vi "PH_Beckhoff-16BB_Testtool.panel.vi"(0 "object ref":refnum<vi>, 5 "error in (no error)":errorcluster) -> (19 "error out":errorcluster)   [LabVIEW 2014, in "PH_Beckhoff-16BB_Testtool.lvlib"]
doc: "By this VI a ross relais can be monitored and switched. \n\nThe indicators \"CLOSED\", \"OPEN\" and \"SWITCH STATE\" show the value of the Beckhoff-Tag: blue indicates bad tag status reference problems, darkgreen false and lightgreen on. If everything is working fine, \"CLOSED\" and \"SWITCH STATE\" should show the same value, while \"OPEN\" has the opposite value. \n\nThe oval button switches the ross relais. It should be in the same state as the \"SWITCH STATE\" indicator. \n\n\"EXIT\" closes the front panel (GUI), while \"Delete Instance\" disconnects and removes the instance from the PCS.\n\nThis VI has no machine safety relevant logig: there is neither a check of internal conclict nor with other objects, for example conflict with other ross relais. Therefore it must be handled with care and should be operated by well educated operators only. It is forseen exclusively for direct operating and testing of the system. \n\nLicense Agreement for this software:\n\nCopyright (C)\nGesellschaft für Schwerionenforschung, GSI\nPlanckstr. 1\n64291 Darmstadt\nGermany\n\nContact: D.Beck@gsi.de \n\nThis program is free software; you can redistribute it and/or modify it under the terms of the GNU General Public License as published by the Free Software Foundation; either version 2 of the license, or (at your option) any later version.\n\nThis program is distributed in the hope that it will be useful, but WITHOUT ANYW ARRANTY; without even the implied warranty of MERCHANTABILITY or FITNESS FOR A PARTICULAR PURPOSE. See the GNU General License for more details (http://www.gnu.org).\n\nGesellschaft für Schwerionenforschung, GSI\nPlanckstr. 1, 64291 Darmstadt, Germany\nFor all questions and ideas contact: M.Richter@gsi.de, H.Brand@gsi.de or D.Beck@gsi.de.\nLast update: 18-DEC-2002"
uses:
  PH_Beckhoff-16BB_Testtool.lvlib
  CS_Core/CSSystem/CoreLib/CoreLib.short 2 byte array.vi
  CS_Core/CSSystem/CoreLib/CoreLib.string 2 byte array.vi
  PH_Basics/PH_Common/PH_Common.lvlib
  CS_Core/BaseProcess/BaseProcess.lvlib
  CS_Core/CSSystem/CoreLib/CoreLib.lvlib
  PH_Basics/PH_Class/PH_Class.lvlib
panel:
  out "Instance":string
  out "_DC_int_ok":u32(colorbox) caption="POWER Int"
  in  "Move in 16":bool caption="Dir"
  in  "Move 16":bool caption="Move"
  out "_BB_16_remote_controlled":u32(colorbox) caption="REMOTE"
  out "_BB_16_out":u32(colorbox) caption="OUT"
  out "_BB_16_in":u32(colorbox) caption="IN"
  out "_BB_16_move":u32(colorbox) caption="MOVE"
  out "_BB_16_move_in":u32(colorbox) caption="MOVE IN"
  in  "Move in 15":bool caption="Dir"
  in  "Move 15":bool caption="Move"
  out "_BB_15_remote_controlled":u32(colorbox) caption="REMOTE"
  out "_BB_15_out":u32(colorbox) caption="OUT"
  out "_BB_15_in":u32(colorbox) caption="IN"
  out "_BB_15_move":u32(colorbox) caption="MOVE"
  out "_BB_15_move_in":u32(colorbox) caption="MOVE IN"
  in  "Move in 14":bool caption="Dir"
  in  "Move 14":bool caption="Move"
  out "_BB_14_remote_controlled":u32(colorbox) caption="REMOTE"
  out "_BB_14_out":u32(colorbox) caption="OUT"
  out "_BB_14_in":u32(colorbox) caption="IN"
  out "_BB_14_move":u32(colorbox) caption="MOVE"
  out "_BB_14_move_in":u32(colorbox) caption="MOVE IN"
  in  "Move in 13":bool caption="Dir"
  in  "Move 13":bool caption="Move"
  out "_BB_13_remote_controlled":u32(colorbox) caption="REMOTE"
  out "_BB_13_out":u32(colorbox) caption="OUT"
  out "_BB_13_in":u32(colorbox) caption="IN"
  out "_BB_13_move":u32(colorbox) caption="MOVE"
  out "_BB_13_move_in":u32(colorbox) caption="MOVE IN"
  in  "Move in 12":bool caption="Dir"
  in  "Move 12":bool caption="Move"
  out "_BB_12_remote_controlled":u32(colorbox) caption="REMOTE"
  out "_BB_12_out":u32(colorbox) caption="OUT"
  out "_BB_12_in":u32(colorbox) caption="IN"
  out "_BB_12_move":u32(colorbox) caption="MOVE"
  out "_BB_12_move_in":u32(colorbox) caption="MOVE IN"
  in  "Move in 11":bool caption="Dir"
  in  "Move 11":bool caption="Move"
  out "_BB_11_remote_controlled":u32(colorbox) caption="REMOTE"
  out "_BB_11_out":u32(colorbox) caption="OUT"
  out "_BB_11_in":u32(colorbox) caption="IN"
  out "_BB_11_move":u32(colorbox) caption="MOVE"
  out "_BB_11_move_in":u32(colorbox) caption="MOVE IN"
  in  "Move in 10":bool caption="Dir"
  in  "Move 10":bool caption="Move"
  out "_BB_10_remote_controlled":u32(colorbox) caption="REMOTE"
  out "_BB_10_out":u32(colorbox) caption="OUT"
  out "_BB_10_in":u32(colorbox) caption="IN"
  out "_BB_10_move":u32(colorbox) caption="MOVE"
  out "_BB_10_move_in":u32(colorbox) caption="MOVE IN"
  in  "Move in 9":bool caption="Dir"
  in  "Move 9":bool caption="Move"
  out "_BB_9_remote_controlled":u32(colorbox) caption="REMOTE"
  out "_BB_9_out":u32(colorbox) caption="OUT"
  out "_BB_9_in":u32(colorbox) caption="IN"
  out "_BB_9_move":u32(colorbox) caption="MOVE"
  out "_BB_9_move_in":u32(colorbox) caption="MOVE IN"
  in  "Move in 8":bool caption="Dir"
  in  "Move 8":bool caption="Move"
  out "_BB_8_remote_controlled":u32(colorbox) caption="REMOTE"
  out "_BB_8_out":u32(colorbox) caption="OUT"
  out "_BB_8_in":u32(colorbox) caption="IN"
  out "_BB_8_move":u32(colorbox) caption="MOVE"
  out "_BB_8_move_in":u32(colorbox) caption="MOVE IN"
  in  "Move in 7":bool caption="Dir"
  in  "Move 7":bool caption="Move"
  out "_BB_7_remote_controlled":u32(colorbox) caption="REMOTE"
  out "_BB_7_out":u32(colorbox) caption="OUT"
  out "_BB_7_in":u32(colorbox) caption="IN"
  out "_BB_7_move":u32(colorbox) caption="MOVE"
  out "_BB_7_move_in":u32(colorbox) caption="MOVE IN"
  in  "Move in 6":bool caption="Dir"
  in  "Move 6":bool caption="Move"
  out "_BB_6_remote_controlled":u32(colorbox) caption="REMOTE"
  out "_BB_6_out":u32(colorbox) caption="OUT"
  out "_BB_6_in":u32(colorbox) caption="IN"
  out "_BB_6_move":u32(colorbox) caption="MOVE"
  out "_BB_6_move_in":u32(colorbox) caption="MOVE IN"
  in  "Move in 5":bool caption="Dir"
  in  "Move 5":bool caption="Move"
  out "_BB_5_remote_controlled":u32(colorbox) caption="REMOTE"
  out "_BB_5_out":u32(colorbox) caption="OUT"
  out "_BB_5_in":u32(colorbox) caption="IN"
  out "_BB_5_move":u32(colorbox) caption="MOVE"
  out "_BB_5_move_in":u32(colorbox) caption="MOVE IN"
  in  "Move in 4":bool caption="Dir"
  in  "Move 4":bool caption="Move"
  out "_BB_4_remote_controlled":u32(colorbox) caption="REMOTE"
  out "_BB_4_out":u32(colorbox) caption="OUT"
  out "_BB_4_in":u32(colorbox) caption="IN"
  out "_BB_4_move":u32(colorbox) caption="MOVE"
  out "_BB_4_move_in":u32(colorbox) caption="MOVE IN"
  in  "Move in 3":bool caption="Dir"
  in  "Move 3":bool caption="Move"
  out "_BB_3_remote_controlled":u32(colorbox) caption="REMOTE"
  out "_BB_3_out":u32(colorbox) caption="OUT"
  out "_BB_3_in":u32(colorbox) caption="IN"
  out "_BB_3_move":u32(colorbox) caption="MOVE"
  out "_BB_3_move_in":u32(colorbox) caption="MOVE IN"
  in  "Move in 2":bool caption="Dir"
  in  "Move 2":bool caption="Move"
  out "_BB_2_remote_controlled":u32(colorbox) caption="REMOTE"
  out "_BB_2_out":u32(colorbox) caption="OUT"
  out "_BB_2_in":u32(colorbox) caption="IN"
  out "_BB_2_move":u32(colorbox) caption="MOVE"
  out "_BB_2_move_in":u32(colorbox) caption="MOVE IN"
  out "_DC_ext_ok":u32(colorbox) caption="POWER Ext"
  in  "Move in 1":bool caption="Dir"
  in  "Move 1":bool caption="Move"
  out "_BB_1_remote_controlled":u32(colorbox) caption="REMOTE"
  out "_BB_1_out":u32(colorbox) caption="OUT"
  out "_BB_1_in":u32(colorbox) caption="IN"
  out "_BB_1_move":u32(colorbox) caption="MOVE"
  out "_BB_1_move_in":u32(colorbox) caption="MOVE IN"
  in  "Delete":bool
  # "PCS"
  # "3.40"
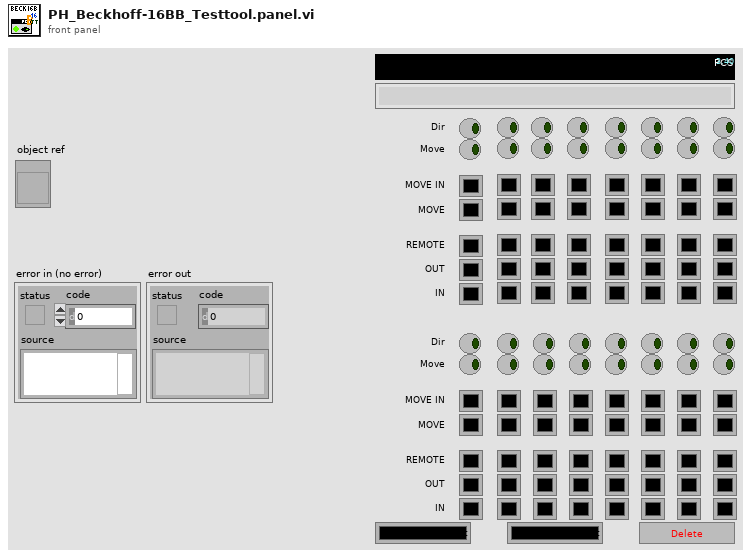
[diagram p1: front panel]
types:
  T1 = typedef "PH_Beckhoff-16BB_Testtool.lvlib/PH_Beckhoff-16BB_Testtool.i attribute.ctl" = cluster{"GUI Refs":refnum<vi>[], "16BB Instance":string}
  T2 = typedef "CoreDefs.rawDataType.ctl" = i8[]
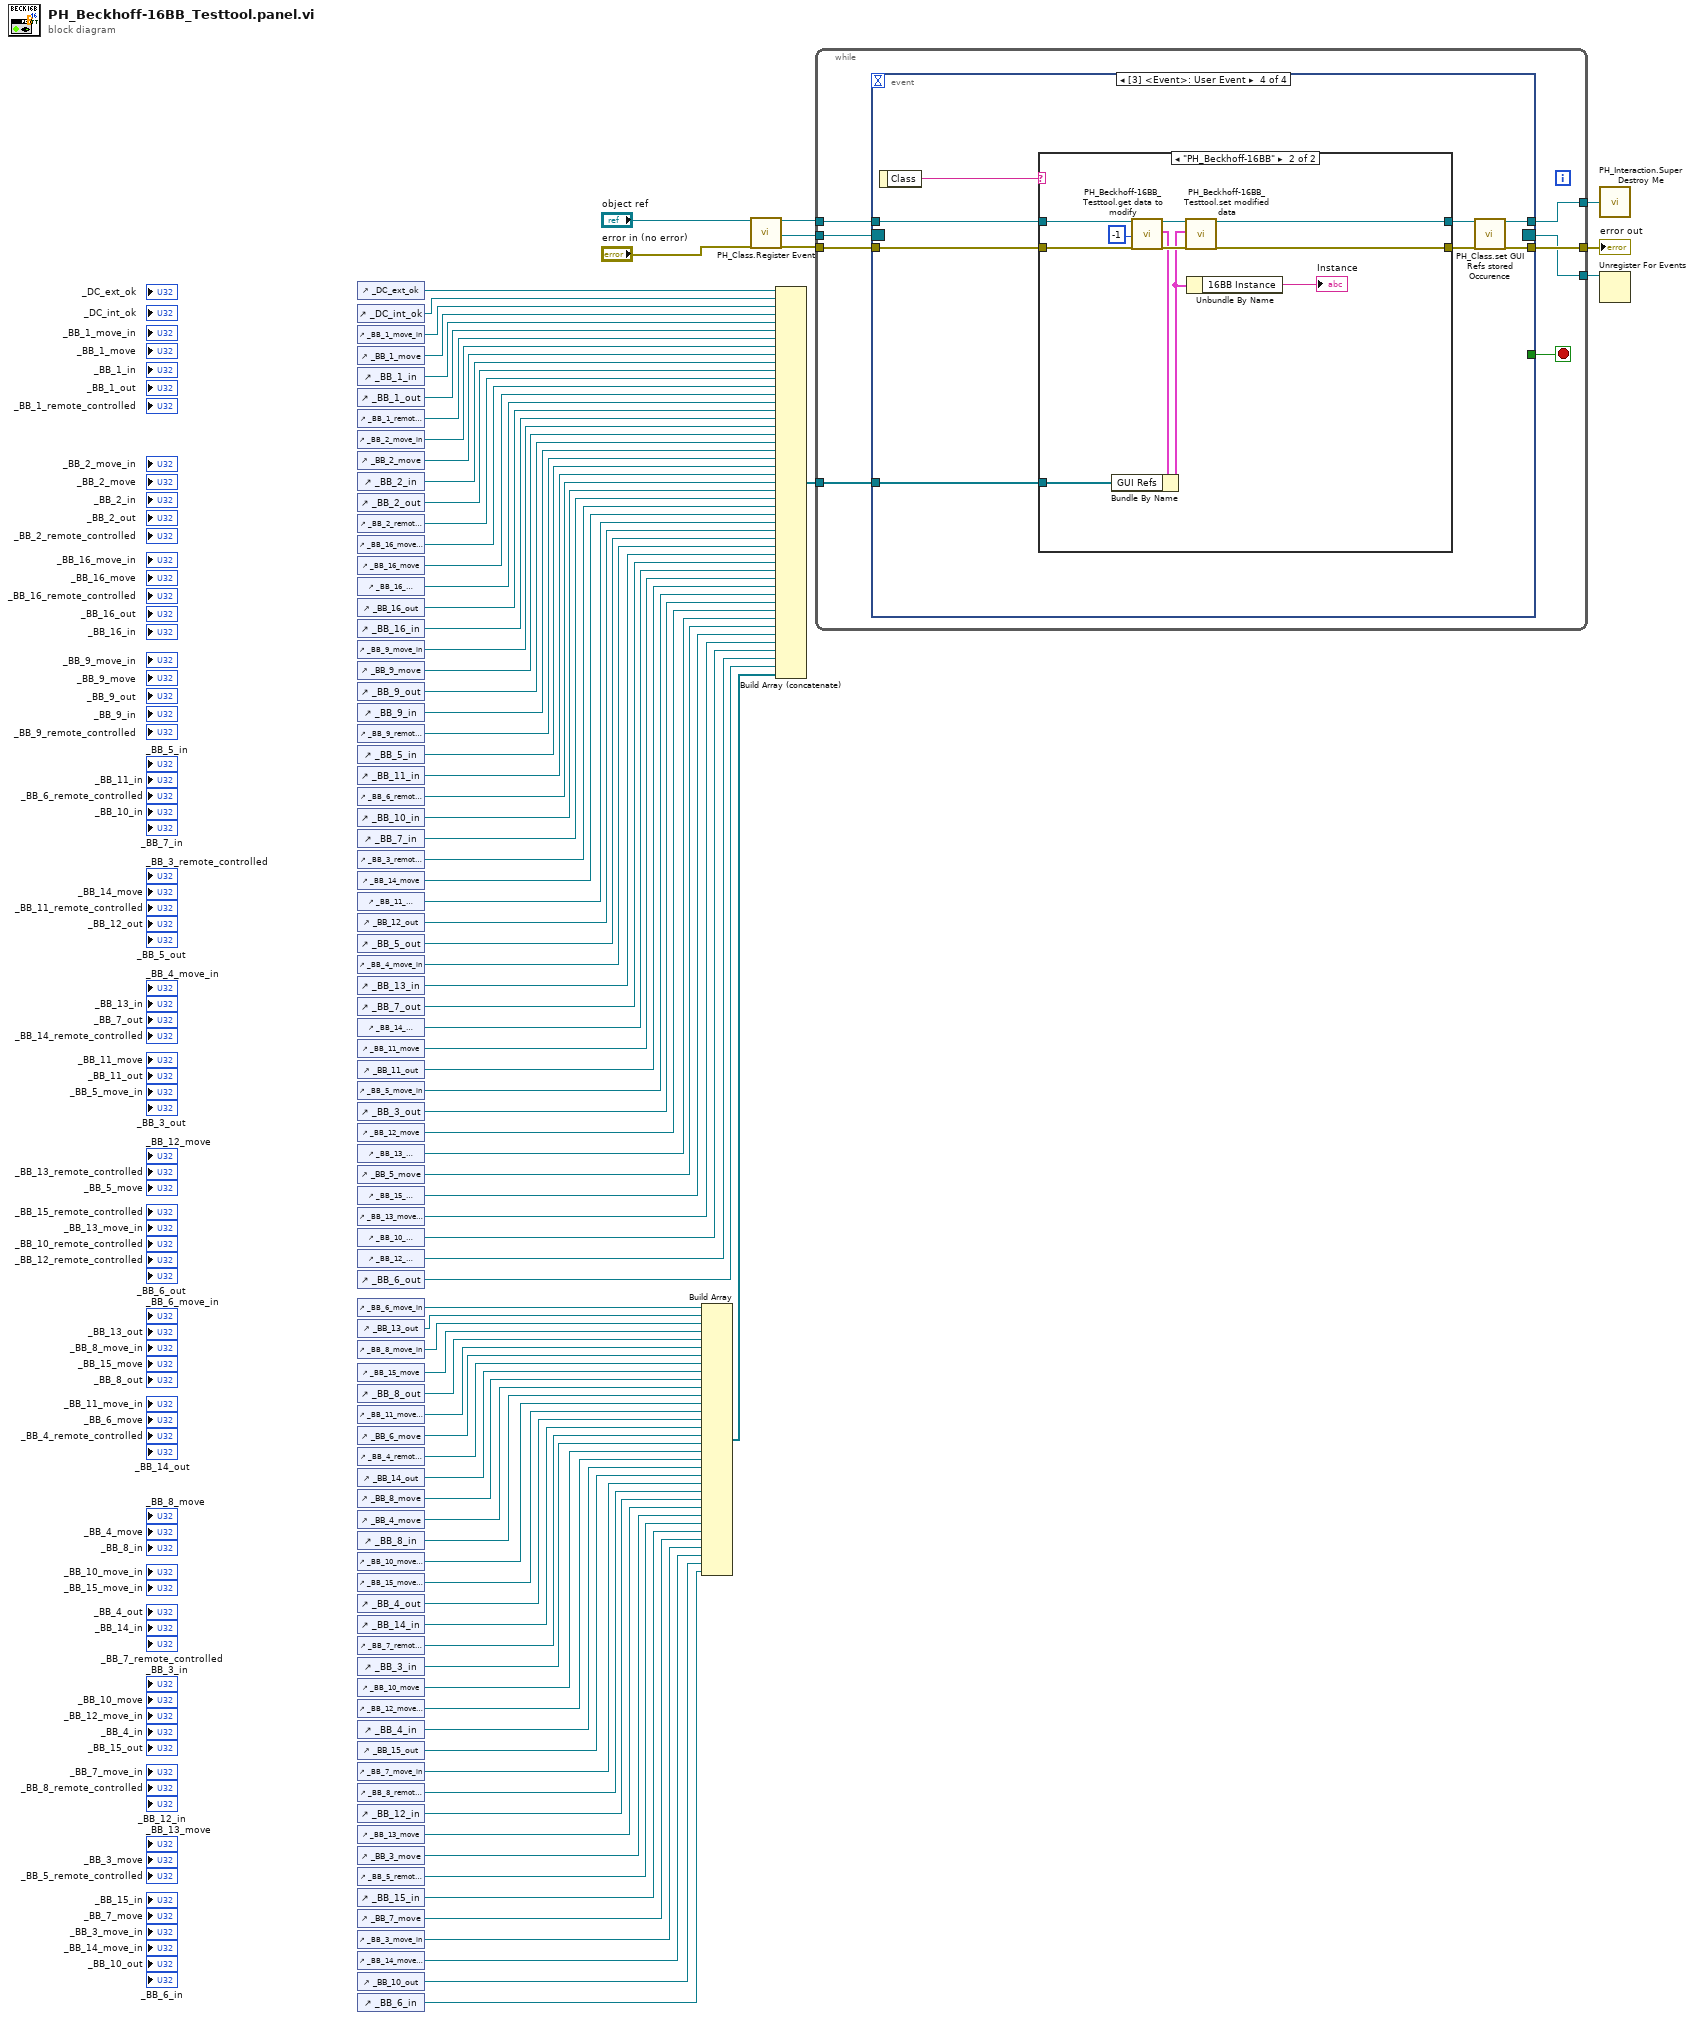
[diagram p0: block diagram]
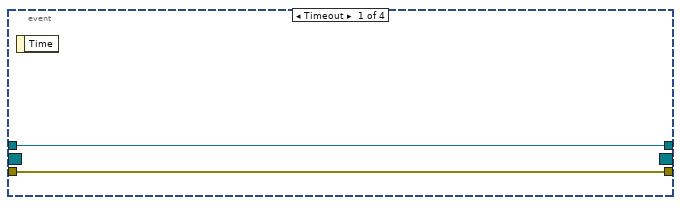
[diagram p2: hidden frame]
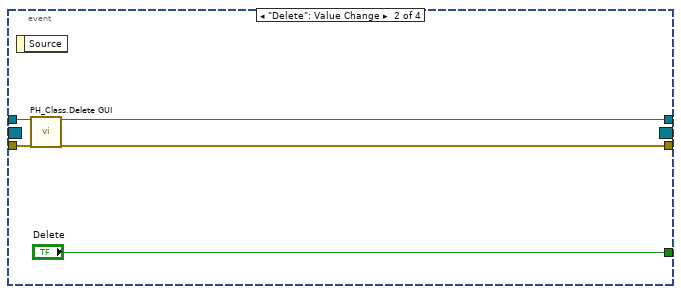
[diagram p3: hidden frame]
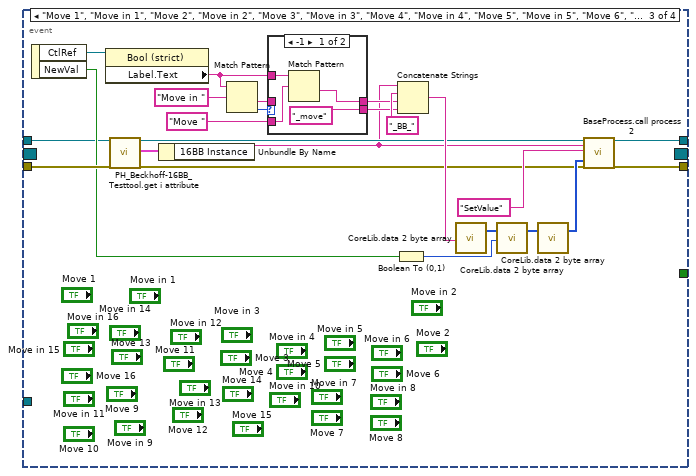
[diagram p4: hidden frame]
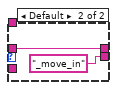
[diagram p5: hidden frame]
diagram:
  n1 = control-ref of="_DC_ext_ok"() -> (w84:refnum<vi>)
  n2 = control-ref of="_DC_int_ok"() -> (w85:refnum<vi>)
  n3 = control-ref of="_BB_1_move_in"() -> (w90:refnum<vi>)
  n4 = control-ref of="_BB_1_move"() -> (w89:refnum<vi>)
  n5 = control-ref of="_BB_1_in"() -> (w88:refnum<vi>)
  n6 = control-ref of="_BB_1_out"() -> (w87:refnum<vi>)
  n7 = control-ref of="_BB_1_remote_controlled"() -> (w86:refnum<vi>)
  n8 = control-ref of="_BB_2_move_in"() -> (w83:refnum<vi>)
  n9 = control-ref of="_BB_2_move"() -> (w82:refnum<vi>)
  n10 = control-ref of="_BB_2_in"() -> (w81:refnum<vi>)
  n11 = control-ref of="_BB_2_out"() -> (w80:refnum<vi>)
  n12 = control-ref of="_BB_2_remote_controlled"() -> (w79:refnum<vi>)
  n13 = control-ref of="_BB_16_move_in"() -> (w78:refnum<vi>)
  n14 = control-ref of="_BB_16_move"() -> (w77:refnum<vi>)
  n15 = control-ref of="_BB_16_remote_controlled"() -> (w76:refnum<vi>)
  n16 = control-ref of="_BB_16_out"() -> (w75:refnum<vi>)
  n17 = control-ref of="_BB_16_in"() -> (w74:refnum<vi>)
  n18 = control-ref of="_BB_9_move_in"() -> (w73:refnum<vi>)
  n19 = control-ref of="_BB_9_move"() -> (w72:refnum<vi>)
  n20 = control-ref of="_BB_9_out"() -> (w71:refnum<vi>)
  n21 = control-ref of="_BB_9_in"() -> (w70:refnum<vi>)
  n22 = control-ref of="_BB_9_remote_controlled"() -> (w69:refnum<vi>)
  n23 = control-ref of="_BB_5_in"() -> (w68:refnum<vi>)
  n24 = control-ref of="_BB_11_in"() -> (w67:refnum<vi>)
  n25 = control-ref of="_BB_6_remote_controlled"() -> (w66:refnum<vi>)
  n26 = control-ref of="_BB_10_in"() -> (w65:refnum<vi>)
  n27 = control-ref of="_BB_7_in"() -> (w64:refnum<vi>)
  n28 = control-ref of="_BB_3_remote_controlled"() -> (w63:refnum<vi>)
  n29 = control-ref of="_BB_14_move"() -> (w62:refnum<vi>)
  n30 = control-ref of="_BB_11_remote_controlled"() -> (w61:refnum<vi>)
  n31 = control-ref of="_BB_12_out"() -> (w60:refnum<vi>)
  n32 = control-ref of="_BB_5_out"() -> (w59:refnum<vi>)
  n33 = control-ref of="_BB_4_move_in"() -> (w58:refnum<vi>)
  n34 = control-ref of="_BB_13_in"() -> (w57:refnum<vi>)
  n35 = control-ref of="_BB_7_out"() -> (w56:refnum<vi>)
  n36 = control-ref of="_BB_14_remote_controlled"() -> (w55:refnum<vi>)
  n37 = control-ref of="_BB_11_move"() -> (w54:refnum<vi>)
  n38 = control-ref of="_BB_11_out"() -> (w53:refnum<vi>)
  n39 = control-ref of="_BB_5_move_in"() -> (w52:refnum<vi>)
  n40 = control-ref of="_BB_3_out"() -> (w51:refnum<vi>)
  n41 = control-ref of="_BB_12_move"() -> (w50:refnum<vi>)
  n42 = control-ref of="_BB_13_remote_controlled"() -> (w49:refnum<vi>)
  n43 = control-ref of="_BB_5_move"() -> (w48:refnum<vi>)
  n44 = control-ref of="_BB_15_remote_controlled"() -> (w47:refnum<vi>)
  n45 = control-ref of="_BB_13_move_in"() -> (w46:refnum<vi>)
  n46 = control-ref of="_BB_10_remote_controlled"() -> (w45:refnum<vi>)
  n47 = control-ref of="_BB_12_remote_controlled"() -> (w44:refnum<vi>)
  n48 = control-ref of="_BB_6_out"() -> (w43:refnum<vi>)
  n49 = control-ref of="_BB_6_move_in"() -> (w42:refnum<vi>)
  n50 = control-ref of="_BB_13_out"() -> (w41:refnum<vi>)
  n51 = control-ref of="_BB_8_move_in"() -> (w40:refnum<vi>)
  n52 = control-ref of="_BB_15_move"() -> (w39:refnum<vi>)
  n53 = control-ref of="_BB_8_out"() -> (w38:refnum<vi>)
  n54 = control-ref of="_BB_11_move_in"() -> (w37:refnum<vi>)
  n55 = control-ref of="_BB_6_move"() -> (w36:refnum<vi>)
  n56 = control-ref of="_BB_4_remote_controlled"() -> (w35:refnum<vi>)
  n57 = control-ref of="_BB_14_out"() -> (w34:refnum<vi>)
  n58 = control-ref of="_BB_8_move"() -> (w32:refnum<vi>)
  n59 = control-ref of="_BB_4_move"() -> (w31:refnum<vi>)
  n60 = control-ref of="_BB_8_in"() -> (w30:refnum<vi>)
  n61 = control-ref of="_BB_10_move_in"() -> (w29:refnum<vi>)
  n62 = control-ref of="_BB_15_move_in"() -> (w28:refnum<vi>)
  n63 = control-ref of="_BB_4_out"() -> (w27:refnum<vi>)
  n64 = control-ref of="_BB_14_in"() -> (w26:refnum<vi>)
  n65 = control-ref of="_BB_7_remote_controlled"() -> (w25:refnum<vi>)
  n66 = control-ref of="_BB_3_in"() -> (w24:refnum<vi>)
  n67 = control-ref of="_BB_10_move"() -> (w23:refnum<vi>)
  n68 = control-ref of="_BB_12_move_in"() -> (w22:refnum<vi>)
  n69 = control-ref of="_BB_4_in"() -> (w21:refnum<vi>)
  n70 = control-ref of="_BB_15_out"() -> (w20:refnum<vi>)
  n71 = control-ref of="_BB_7_move_in"() -> (w19:refnum<vi>)
  n72 = control-ref of="_BB_8_remote_controlled"() -> (w18:refnum<vi>)
  n73 = control-ref of="_BB_12_in"() -> (w17:refnum<vi>)
  n74 = control-ref of="_BB_13_move"() -> (w16:refnum<vi>)
  n75 = control-ref of="_BB_3_move"() -> (w15:refnum<vi>)
  n76 = control-ref of="_BB_5_remote_controlled"() -> (w14:refnum<vi>)
  n77 = control-ref of="_BB_15_in"() -> (w13:refnum<vi>)
  n78 = control-ref of="_BB_7_move"() -> (w12:refnum<vi>)
  n79 = control-ref of="_BB_3_move_in"() -> (w11:refnum<vi>)
  n80 = control-ref of="_BB_14_move_in"() -> (w10:refnum<vi>)
  n81 = control-ref of="_BB_10_out"() -> (w9:refnum<vi>)
  n82 = control-ref of="_BB_6_in"() -> (w8:refnum<vi>)
  n83 = Build Array(w42, w41, w40, w39, w38, w37, w36, w35, w34, w32, w31, w30, w29, w28, w27, w26, w25, w24, w23, w22, w21, w20, w19, w18, w17, w16, w15, w14, w13, w12, w11, w10, w9, w8) -> (w33:refnum<vi>[])
  n84 = call "PH_Class.Register Event.vi"("i ref in"="object ref", "error in (no error)"="error in (no error)") -> ("i ref out"=w7:refnum<vi>, "Event Registration Refnum"=w5:refnum<event-registration>, "error out"=w6:errorcluster)  [unwired: 15 in]
  n85 = Build Array (concatenate)(w84, w85, w90, w89, w88, w87, w86, w83, w82, w81, w80, w79, w78, w77, w76, w75, w74, w73, w72, w71, w70, w69, w68, w67, w66, w65, w64, w63, w62, w61, w60, w59, w58, w57, w56, w55, w54, w53, w52, w51, w50, w49, w48, w47, w46, w45, w44, w43, w33) -> (w3:refnum<vi>[])
  n86 = while {
    tunnel: w7 -> [w97]
    tunnel: [w96] -> w92
    tunnel: w6 -> [w99]
    tunnel: [w98] -> w91
    tunnel: w5 -> [w95]
    tunnel: [w94] -> w4
    tunnel: w3 -> [w93]
    stop <- w100 stop-if-true
    n87 = event shown="[3] <Event>: User Event" {
      selector: w95 -> [_ _ _ _]
      dyn-events: [_ _ _ _] -> w94
      timeout: _ -> [_ _ _ _]
      tunnel: [_ "Delete" _ _] -> w100
      tunnel: w97 -> [w101 w106 w111 w143]
      tunnel: w99 -> [w102 w105 w130 w141]
      tunnel: [w102 w104 w129 w144] -> w98
      tunnel: [w101 w103 w131 w145] -> w96
      tunnel: w93 -> [_ _ _ w138]
      event Timeout {
        n88 = event-data() -> ()  [unwired: 1 in, 1 out]
      }
      event "Delete": Value Change {
        n89 = event-data() -> ()  [unwired: 1 in, 1 out]
        n90 = call "PH_Class.Delete GUI.vi"("VI in"=w106, "error in (no error)"=w105) -> ("VI out"=w103:refnum<vi>, "error out"=w104:errorcluster)  [unwired: 16 in]
      }
      event "Move 1", "Move in 1", "Move 2", "Move in 2", "Move 3", "Move in 3", "Move 4", "Move in 4", "Move 5", "Move in 5", "Move 6", "Move in 6", "Move 7", "Move in 7", "Move 8", "Move in 8", "Move 9", "Move in 9", "Move 10", "Move in 10", "Move 11", "Move in 11", "Move 12", "Move in 12", "Move 13", "Move in 13", "Move 14", "Move in 14", "Move 15", "Move in 15", "Move 16", "Move in 16": Value Change {
        n91 = event-data() -> ("CtlRef"=w128:refnum<vi>, "NewVal"=w118:bool)  [unwired: 1 in]
        n92 = property class="Bool (strict)"(reference=w128) -> ("Label.Text"=w116:string)  [unwired: 1 in, 2 out]
        n93 = call "PH_Beckhoff-16BB_Testtool.get i attribute.vi"("i ref in"=w111, "error in (no error)"=w130) -> ("i ref out"=w110:refnum<vi>, "i attribute"=w109:T1, "error out"=w112:errorcluster)  [unwired: 15 in]
        n94 = Unbundle By Name(w109) -> ("16BB Instance"=w108:string)
        n95 = Match Pattern(string=w116, regular expression="Move in ") -> (after substring=w125:string, offset past match=w126:i32)  [unwired: 1 in, 2 out]
        n96 = case shown="-1" w126 {
          tunnel: w125 -> [_ w137]
          tunnel: [w133 w137] -> w123
          tunnel: ["_move" "_move_in"] -> w122
          tunnel: w116 -> [w135 _]
          tunnel: "Move " ("regular expression") -> [w134 _]
          frame -1 {
            n97 = Match Pattern(string=w135, regular expression=w134) -> (after substring=w133:string)  [unwired: 1 in, 3 out]
          }
          frame Default {
          }
        }
        n98 = Boolean To (0,1)(Boolean=w118) -> (0, 1=w117:i16)
        n99 = Concatenate Strings(w108, "_BB_" ("string"), w123, w122) -> (w120:string)
        n100 = call-poly "CoreLib.data 2 byte array.vi"("string"=w120) -> ("byteArray out"=w119:T2)  [unwired: 18 in]
        n101 = call-poly "CoreLib.data 2 byte array.vi"("byteArray"=w119, "i16"=w117) -> ("byteArray out"=w114:T2)  [unwired: 17 in]
        n102 = call-poly "CoreLib.data 2 byte array.vi"("byteArray"=w114) -> ("byteArray out"=w113:T2)  [unwired: 18 in]
        n103 = call "BaseProcess.call process 2.vi"("i ref in"=w110, "Object"=w108, "Selector"="SetValue" ("string"), "Data"=w113, "error in (no error)"=w112) -> ("i ref out"=w131:refnum<vi>, "error out"=w129:errorcluster)  [unwired: 13 in]
      }
      event User Event {
        n104 = event-data() -> ("Class"=w139:string)  [unwired: 1 in]
        n105 = case shown="\"PH_Beckhoff-16BB\"" w139 {
          tunnel: w143 -> [w147 w154]
          tunnel: [w147 w153] -> w142
          tunnel: w141 -> [w146 w152]
          tunnel: [w146 w151] -> w140
          tunnel: w138 -> [_ w150]
          frame Default {
          }
          frame "PH_Beckhoff-16BB" {
            n106 = call "PH_Beckhoff-16BB_Testtool.get data to modify.vi"("i ref in"=w154, "ms timeout (10000)"=-1, "error in (no error)"=w152) -> ("i ref out"=w158:refnum<vi>, "i attribute"=w156:T1, "error out"=w157:errorcluster)  [unwired: 13 in, 1 out]
            n107 = Bundle By Name(cluster=w156, "GUI Refs"=w150) -> (w149:T1)
            n108 = call "PH_Beckhoff-16BB_Testtool.set modified data.vi"("i ref in"=w158, "i attribute"=w149, "error in (no error)"=w157) -> ("i ref out"=w153:refnum<vi>, "error out"=w151:errorcluster)  [unwired: 15 in]
            n109 = Unbundle By Name(w149) -> ("16BB Instance"=→"Instance":string)
          }
        }
        n110 = call "PH_Class.set GUI Refs stored Occurence.vi"("i ref in"=w142, "error in (no error)"=w140) -> ("i ref out"=w145:refnum<vi>, "error out"=w144:errorcluster)  [unwired: 16 in]
      }
    }
  }
  "error out" <- w91
  n111 = call "PH_Interaction.Super Destroy Me.vi"("i ref out"=w92) -> ()
  n112 = Unregister For Events(event registration refnum=w4) -> ()  [unwired: 1 in, 1 out]
